vi "DefaultFromIni.vi"(8 "error in (no error)":errorcluster, 11 "SpecAnPlugins.lvlib":refnum<class "Keysight44xx.lvclass">) -> (0 "error out":errorcluster, 3 "SpecAnPlugins.lvlib":refnum<class "Keysight44xx.lvclass">)   [LabVIEW 2018, in "SpecAnPlugins.lvlib" / "Keysight44xx.lvclass"]
doc: "This VI loads the configuration previously stored into INI file for future acquisitions and generations."
uses:
  Keysight44xx.lvclass
  C:/Program Files (x86)/National Instruments/LabVIEW 2018/user.lib/NIST/BaseClasses/BasePlugin_class/BasePlugin.lvclass
  TypeDefs/RFBurst.ctl
  TypeDefs/TV.ctl
  <userlib>/NIST/BaseClasses/BasePlugin_class/BasePlugin.lvclass/BasePlugin.ctl
  <userlib>/NIST/BaseClasses/BasePlugin_class/Accessors/Read PluginIniFilePath.vi
  SpecAnBaseClass/SpecAnBase.lvclass
  <vilib>/Utility/config.llb/NI_LVConfig.lvlib
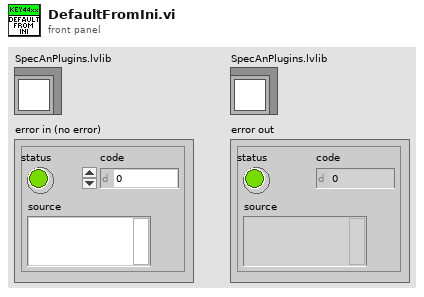
[diagram p1: front panel]
types:
  T1 = typedef "SpecAnPlugins.lvlib/Keysight44xx.lvclass/TV.ctl" = cluster{"Monitor Enabled (OFF)":bool, "SynchronizeSweep":bool, "SynchronizationLineNumber":i32, "TV Field (Any Field)":i32, "TV Signal Format (NTSC-M)":i32, "Trigger Source (Spectrum Analyzer)":i32}
  T2 = typedef "SpecAnPlugins.lvlib/Keysight44xx.lvclass/RFBurst.ctl" = cluster{"Frequency Selectivity (OFF)":bool, "Trigger Level Type (Absolute)":i32, "Narrow Pulse Discriminator (OFF)":bool}
  T3 = typedef "NI_LVConfig.lvlib/Config Data RefNum.ctl" = refnum<k1>
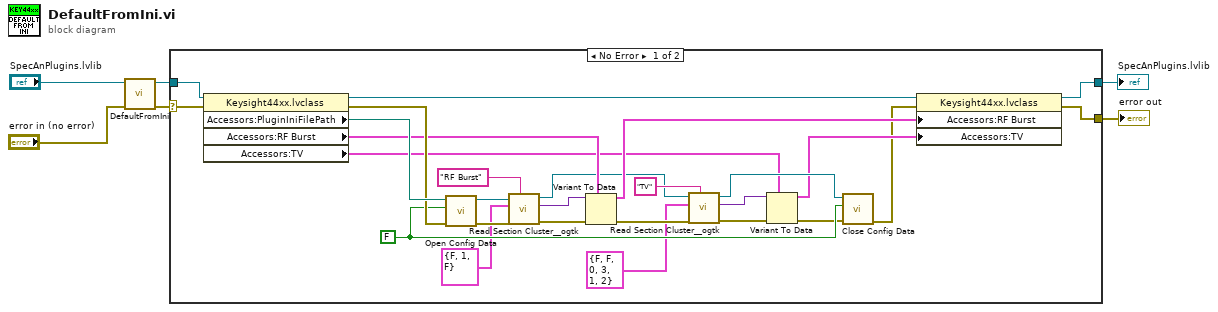
[diagram p0: block diagram]
diagram:
  n1 = call-parent "DefaultFromIni.vi"("error in (no error)"="error in (no error)", "SpecAnPlugins.lvlib"="SpecAnPlugins.lvlib") -> ("error out"=w3:errorcluster, "SpecAnPlugins.lvlib"=w4:refnum<class "Keysight44xx.lvclass">)  [unwired: 8 in]
  n2 = case shown="No Error" w3 {
    selector: w3 -> [w32 w34]
    tunnel: w4 -> [w33 w35]
    tunnel: [w20 w35] -> w2
    tunnel: [w7 w34] -> w1
    frame No Error {
      w24 = FALSE ("create file if necessary (T)")
      n3 = property class="Keysight44xx.lvclass"(reference=w33, error in=w32) -> (reference out=w21:refnum<class "Keysight44xx.lvclass">, error out=w30:errorcluster, "Accessors:PluginIniFilePath"=w31:path, "Accessors:RF Burst"=w23:T2, "Accessors:TV"=w10:T1)
      n4 = call <vilib>:"Open Config Data.vi"("error in (no error)"=w30, "create file if necessary (T)"=w24, "configuration file path"=w31) -> ("error out"=w25:errorcluster, "refnum"=w26:T3)  [unwired: 6 in, 1 out]
      n5 = call <userlib>:"Read Section Cluster__ogtk.vi"("section (optional)"="RF Burst", "error in (no error)"=w25, "Section Formatted Cluster Type"=T2 {"Frequency Selectivity (OFF)"=FALSE, "Trigger Level Type (Absolute)"=1, "Narrow Pulse Discriminator (OFF)"=FALSE} ("RF Burst"), "refnum"=w26) -> ("error out"=w28:errorcluster, "Section Formatted Cluster"=w27:variant, "dup refnum"=w16:T3)  [unwired: 3 in, 2 out]
      n6 = Variant To Data(error in=w28, type=w23, Variant=w27) -> (data=w19:T2, error out=w17:errorcluster)
      n7 = call <userlib>:"Read Section Cluster__ogtk.vi"("section (optional)"="TV", "error in (no error)"=w17, "Section Formatted Cluster Type"=T1 {"Monitor Enabled (OFF)"=FALSE, "SynchronizeSweep"=FALSE, "SynchronizationLineNumber"=0, "TV Field (Any Field)"=3, "TV Signal Format (NTSC-M)"=1, "Trigger Source (Spectrum Analyzer)"=2} ("TV"), "refnum"=w16) -> ("error out"=w14:errorcluster, "Section Formatted Cluster"=w11:variant, "dup refnum"=w12:T3)  [unwired: 3 in, 2 out]
      n8 = Variant To Data(error in=w14, type=w10, Variant=w11) -> (data=w9:T1, error out=w13:errorcluster)
      n9 = call <vilib>:"Close Config Data.vi"("error in (no error)"=w13, "write file if changed (T)"=w24, "refnum"=w12) -> ("error out"=w8:errorcluster)  [unwired: 7 in, 1 out]
      n10 = property class="Keysight44xx.lvclass"(reference=w21, error in=w8, "Accessors:RF Burst"=w19, "Accessors:TV"=w9) -> (reference out=w20:refnum<class "Keysight44xx.lvclass">, error out=w7:errorcluster)
    }
    frame Error {
    }
  }
  "error out" <- w1
  "SpecAnPlugins.lvlib" <- w2
